vi "ValueSignalByPath.vi"(0 "VI Reference In":refnum<vi>, 5 "Control Path":string[](array[string]), 7 "Value (Signaling)":variant, 11 "error in":errorcluster) -> (4 "VI Reference Out":refnum<vi>, 15 "error out":errorcluster)   [LabVIEW 2016]
doc: "This VI sets the value of top level controls in other VI"
uses:
  ControlAction/DoValueSignal/DoValueSignal.lvclass
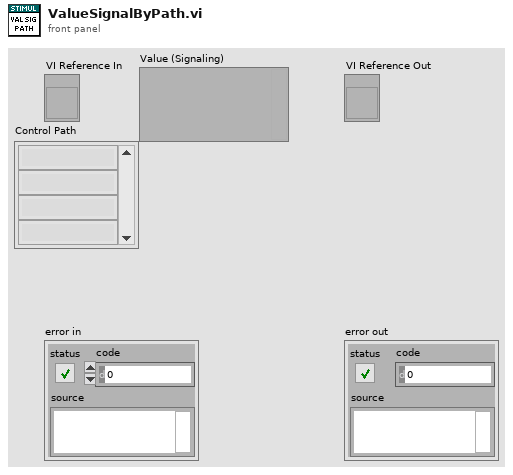
[diagram p1: front panel]
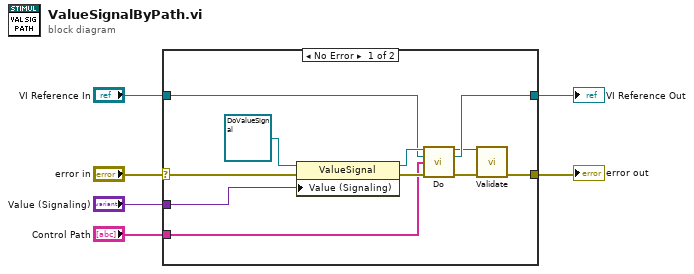
[diagram p0: block diagram]
diagram:
  n1 = case shown="No Error" "error in" {
    selector: "error in" -> [w17 w19]
    tunnel: "Control Path" -> [w13 _]
    tunnel: "VI Reference In" -> [w12 w18]
    tunnel: [w11 w18] -> w3
    tunnel: "Value (Signaling)" -> [w10 _]
    tunnel: [w8 w19] -> w1
    frame No Error {
      n2 = property class="ValueSignal"(reference=refnum<class "DoValueSignal.lvclass"> refnum ("ValueSignal"), error in=w17, "Value (Signaling)"=w10) -> (reference out=w14:refnum<class "DoValueSignal.lvclass">, error out=w16:errorcluster)
      n3 = call-dynamic "Do.vi"("ControlDoBase in"=w14, "VI Reference in"=w12, "Control Path"=w13, "error in"=w16) -> ("ControlDoBase out"=w7:refnum<class "DoValueSignal.lvclass">, "VI Reference out"=w11:refnum<vi>, "error out"=w9:errorcluster)  [unwired: 9 in]
      n4 = call-dynamic "Validate.vi"("ControlDoBase in"=w7, "error in (no error)"=w9) -> ("error out"=w8:errorcluster)  [unwired: 12 in, 1 out]
    }
    frame Error {
    }
  }
  "error out" <- w1
  "VI Reference Out" <- w3
